vi "GLVT-Stepper-RotateDeg.vi"(5 "Pulse Rate (pps)":i32=600, 7 "Steps per Rev":i32=1600, 8 "error in":errorcluster, 9 "Rotate Direction":T1=enum."CW", 10 "Rotation Angle (deg)":dbl min=0.0 max=360.0 step=0.1) -> (0 "error out":errorcluster, 2 "Actual Rotation Angle (deg)":dbl min=0.0 max=360.0 step=0.1)   [LabVIEW 2023]
uses:
  Controls/GLVT-Stepper-RotateDirection.ctl
  Controls/GLVT-Stepper-EnableState.ctl
  <vilib>/DAQmx/write.llb/DAQmx Write (Digital 1D U32 1Chan NSamp).vi
  <vilib>/DAQmx/configure/timing.llb/DAQmx Timing (Sample Clock).vi
  <vilib>/DAQmx/miscellaneous.llb/DAQmx Fill In Error Info.vi
panel:
  out "1/x":dbl format="%^#_2e"
  out "size(s)":i32
  out "Array":u32[](array[numeric])
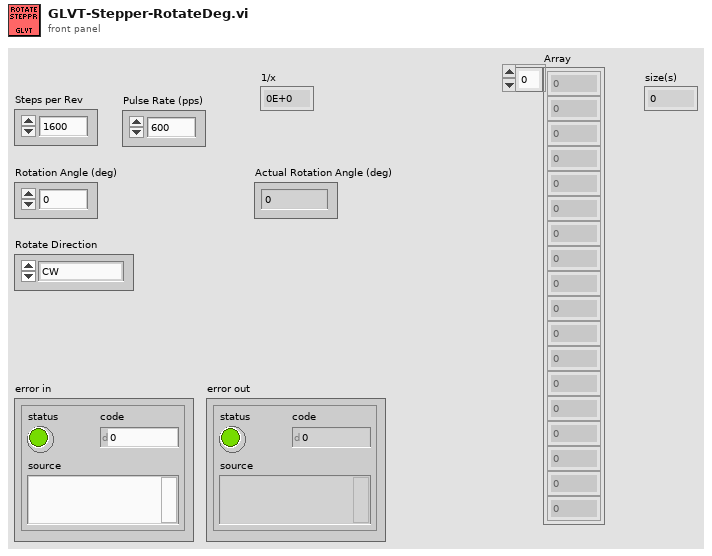
[diagram p1: front panel]
types:
  T1 = typedef "GLVT-Stepper-RotateDirection.ctl" = enum16{"CCW", "CW"}
  T2 = typedef "GLVT-Stepper-EnableState.ctl" = enum16{"Enable", "Disable"}
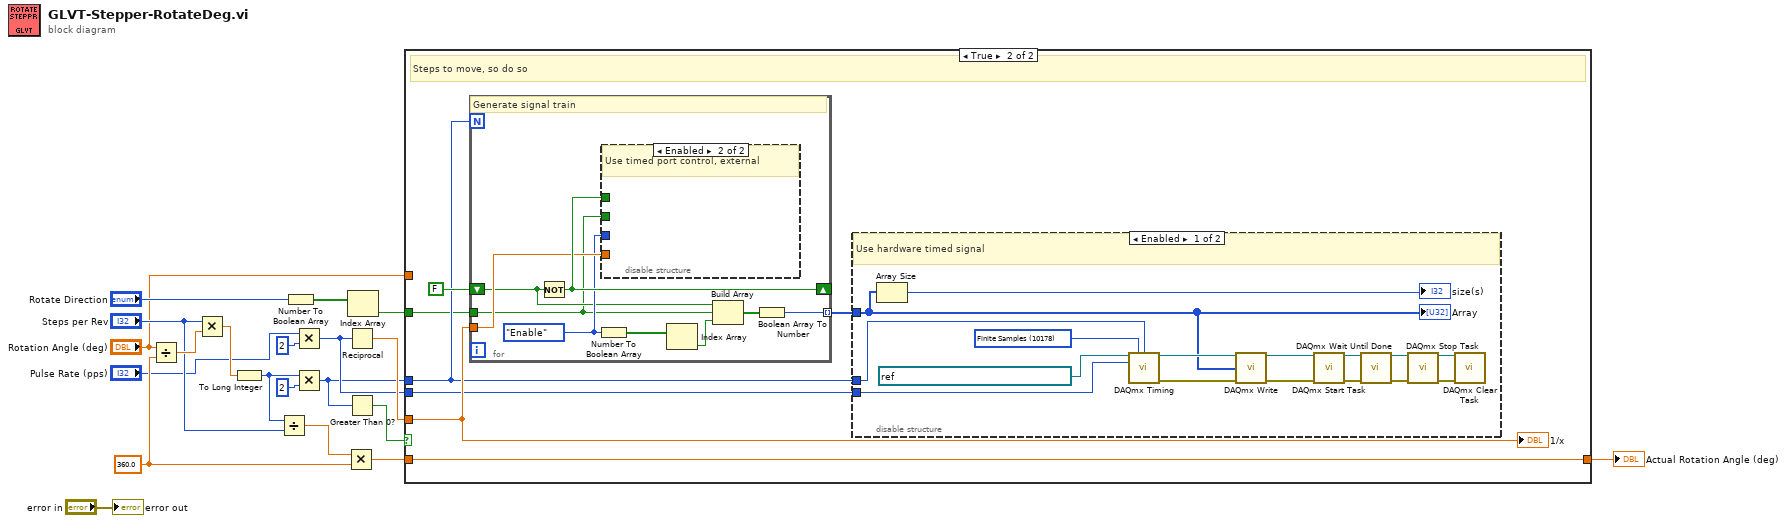
[diagram p0: block diagram]
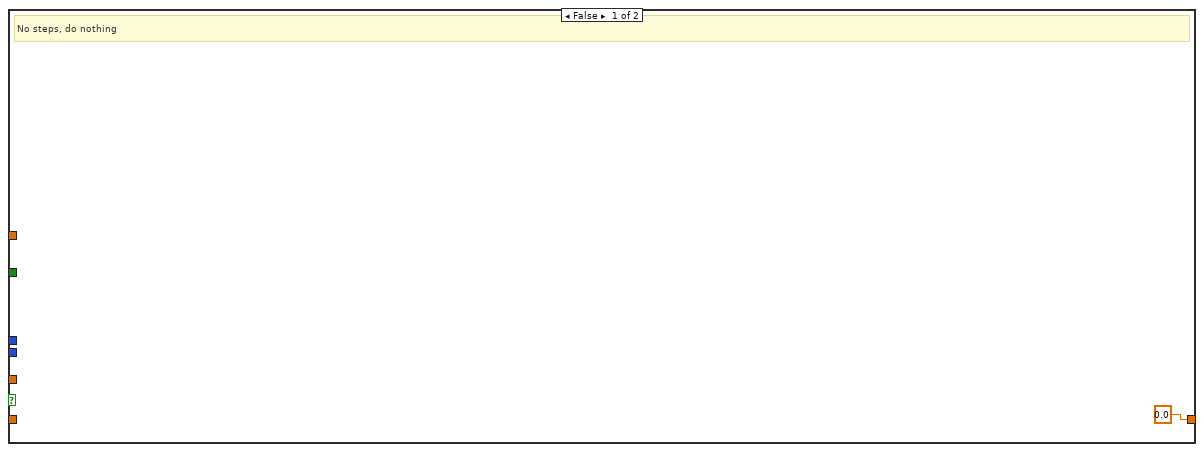
[diagram p2: hidden frame]
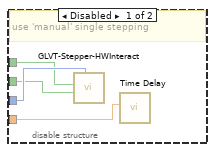
[diagram p4: hidden frame]
diagram:
  w13 = 360.0 ("y")
  n1 = Divide(x="Rotation Angle (deg)", y=w13) -> (x/y=w19:dbl)
  n2 = Multiply(x="Steps per Rev", y=w19) -> (x*y=w18:dbl)
  n3 = To Long Integer(number=w18) -> (32bit integer=w16:i32)
  n4 = Divide(x=w16, y="Steps per Rev") -> (x/y=w14:dbl)
  n5 = Number To Boolean Array(number="Rotate Direction") -> (Boolean array=w8:bool[])
  n6 = Multiply(x="Pulse Rate (pps)", y=2) -> (x*y=w9:i32)
  n7 = Multiply(x=w16, y=2) -> (x*y=w5:i32)
  n8 = Multiply(x=w14, y=w13) -> (x*y=w3:dbl)
  n9 = Reciprocal(x=w9) -> (1/x=w12:dbl)
  n10 = Greater Than 0?(x=w5) -> (x > 0?=w4:bool)
  n11 = Index Array(array=w8) -> (element=w6:bool)  [unwired: 1 in]
  n12 = case shown="True" w4 {
    tunnel: w12 -> [_ w27]
    tunnel: w9 -> [_ w25]
    tunnel: w5 -> [_ w24]
    tunnel: w6 -> [_ w23]
    tunnel: w3 -> [_ w22]
    tunnel: [0.0 w22] -> w2
    tunnel: "Rotation Angle (deg)" -> [_ _]
    frame False {
      # "No steps, do nothing"
    }
    frame True {
      # "Steps to move, so do so"
      n13 = for {
        N: w24 -> [_]
        tunnel: w23 -> [w48]
        shift-right: [w53] -> _
        shift-left: FALSE -> [w49]
        tunnel: w27 -> [w52]
        tunnel: [w45] -> w26 mode=indexing
        w51 = GLVT-Stepper-EnableState."Enable" ("GLVT-Enable State")
        # "Generate signal train"
        n14 = Not(x=w49) -> (.not. x?=w53:bool)
        n15 = Number To Boolean Array(number=w51) -> (Boolean array=w50:bool[])
        n16 = disable-structure shown="Enabled" {
          disable-tunnel: w51 -> [w57 _]
          disable-tunnel: w48 -> [w56 _]
          disable-tunnel: w53 -> [w55 _]
          disable-tunnel: w52 -> [w54 _]
          frame Disabled {
            # "use 'manual' single stepping"
            n17 = call "GLVT-Stepper-HWInteract.vi"("GLVT-Enable State"=w57, "Direction (T=CW)"=w56, "Pulse"=w55) -> ()  [unwired: 8 in, 1 out]
            n18 = call "Time Delay"("Delay Time (s)"=w54) -> ()  [unwired: 10 in, 1 out]
          }
          frame Enabled {
            # "Use timed port control, external"
          }
        }
        n19 = Index Array(array=w50) -> (element=w47:bool)  [unwired: 1 in]
        n20 = Build Array(w49, w48, w47) -> (w46:bool[])
        n21 = Boolean Array To Number(Boolean array=w46) -> (number=w45:u32)
      }
      n22 = disable-structure shown="Enabled" {
        disable-tunnel: w26 -> [w34 _]
        disable-tunnel: w25 -> [w32 _]
        disable-tunnel: w24 -> [w31 _]
        frame Enabled {
          w43 = 10178 items=["Finite Samples"=10178, "Continuous Samples"=10123, "Hardware Timed Single Point"=12522] ("sample mode")
          # "Use hardware timed signal"
          n23 = Array Size(array=w34) -> (size(s)=→"size(s)":i32)
          n24 = call-poly <vilib>:"DAQmx Timing.vi"("task/channels in"=refnum<k21> "GLVT-StepperControlPortMode", "sample mode"=w43, "samples per channel"=w31, "rate"=w32) -> ("task out"=w42:refnum<k21>, "error out"=w35:errorcluster)  [unwired: 10 in]
          n25 = call-poly <vilib>:"DAQmx Write.vi"("task/channels in"=w42, "data"=w34, "error in"=w35) -> ("task out"=w36:refnum<k21>, "error out"=w37:errorcluster)  [unwired: 10 in, 1 out]
          n26 = call <vilib>:"DAQmx Start Task.vi"("task/channels in"=w36, "error in"=w37) -> ("task out"=w38:refnum<k21>, "error out"=w39:errorcluster)  [unwired: 12 in]
          n27 = call <vilib>:"DAQmx Wait Until Done.vi"("task/channels in"=w38, "error in"=w39) -> ("task out"=w40:refnum<k21>, "error out"=w41:errorcluster)  [unwired: 12 in]
          n28 = call <vilib>:"DAQmx Stop Task.vi"("task/channels in"=w40, "error in"=w41) -> ("task out"=w30:refnum<k21>, "error out"=w29:errorcluster)  [unwired: 12 in]
          n29 = call <vilib>:"DAQmx Clear Task.vi"("task in"=w30, "error in"=w29) -> ()  [unwired: 13 in, 1 out]
          "Array" <- w34
        }
        frame Disabled {
          # "Use manual pulse generation"
        }
      }
      "1/x" <- w27
    }
  }
  "Actual Rotation Angle (deg)" <- w2
  "error out" <- "error in"
